vi "Intake_Joint_Set.vi"() -> ()   [LabVIEW 2018]
uses:
  Intake_Joint_Control_Type.ctl
  <vilib>/Rock Robotics/WPI/DriverStation/WPI_DriverStationRobotMode2.ctl
  Intake_Joint_Enum_States.ctl
  Global_Variables/Intake_Joint_Globals.vi
  Global_Variables/Robot_Global_Data.vi
  Global_Variables/Autonomous_Globals.vi
  Global_Variables/Intake_Disc_Globals.vi
panel:
  out "Cargo_Mode_for_Scoring":bool
  out "Cargo_Mode":bool
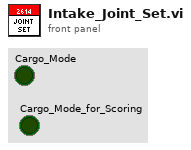
[diagram p1: front panel]
types:
  T1 = typedef "Intake_Joint_Control_Type.ctl" = enum16{"No_Op", "Manual_Joint_Up", "Manual_Joint_Down", "Manual_Position_Control", "Position_Control", "Position"}
  T2 = typedef "WPI_DriverStationRobotMode2.ctl" = enum16{"Autonomous Disabled", "Autonomous Enabled", "Teleop Disabled", "Teleop Enabled", "Disconnected", "Finish", "Test Disabled", "Test Enabled", "Emergency Stopped"}
  T3 = typedef "Intake_Joint_Enum_States.ctl" = enum16{"Current_Position", "High_Rocket_Hatch_Panel_Floor", "High_Rocket_Hatch_Panel", "Mid_Rocket_Hatch_Panel_Floor", "Mid_Rocket_Hatch_Panel", "Low_Rocket_Hatch_Panel", "Cargo_Ship_Hatch_Panel", "Loading_Station_Hatch_Panel", "Ground_Pickup_Hatch_Panel", "High_Rocket_Cargo", "Mid_Rocket_Cargo", "Low_Rocket_Cargo", "Cargo_Ship_Cargo", "Loading_Station_Cargo", "Ground_Pickup_Cargo", "Depot_Pickup_Cargo", "Stow_Cargo", "Get_Hatch"}
  T4 = typedef "Intake_Joint_Notifier.ctl" = cluster{"Intake_Joint_Control_Type":T1, "Manual_Joint_Up":bool, "Manual_Joint_Down":bool, "Low_Rocket":bool, "Mid_Rocket":bool, "High_Rocket":bool, "Cargo_Ship":bool, "Hatch_Floor":bool, "Cargo_Floor":bool, "HP_Hatch":bool, "HP_Cargo":bool, "Depot_Cargo":bool, "Stow":bool, "Intake_Mode":bool, "Set Position":T3, "Parameter_One":dbl, "Parameter_Two":dbl, "Parameter_Three":dbl, "Step":i32, "Joint_Notifier":refnum<notifier>}
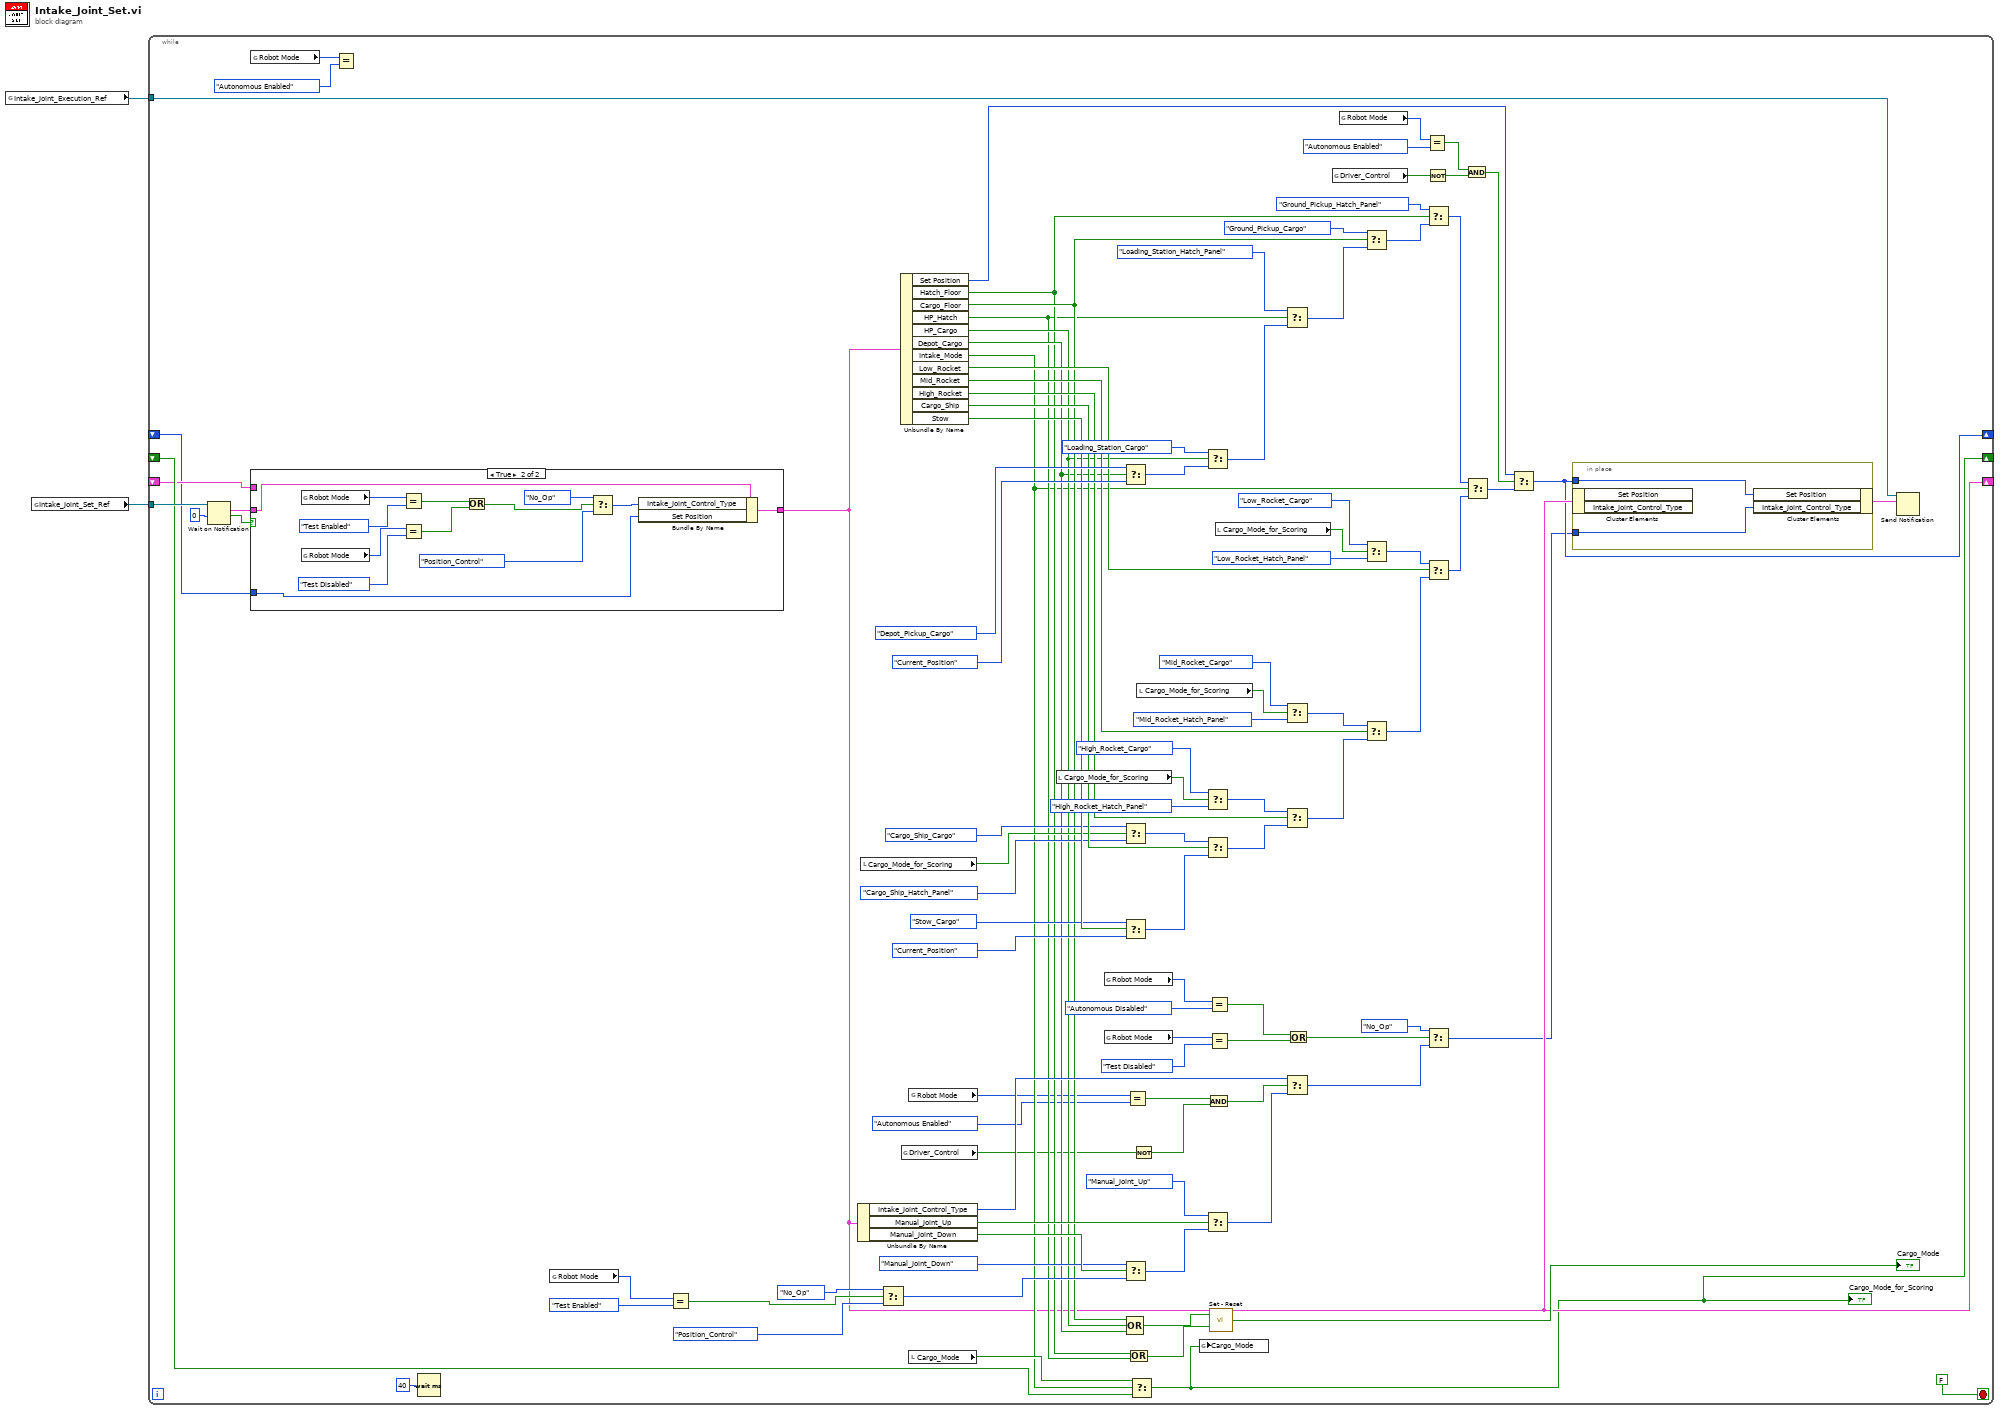
[diagram p0: block diagram]
diagram:
  n1 = global read "Intake_Joint_Globals.vi" "Intake_Joint_Execution_Ref"() -> (w1:refnum<notifier>)
  n2 = global read "Intake_Joint_Globals.vi" "Intake_Joint_Set_Ref"() -> (w2:refnum<notifier>)
  n3 = while {
    tunnel: w2 -> [w102]
    tunnel: w1 -> [w101]
    shift-right: [w23] -> _
    shift-left: _ -> [w36]
    shift-right: [w28] -> _
    shift-left: _ -> [w27]
    shift-right: [w25] -> _
    shift-left: _ -> [w24]
    stop <- FALSE stop-if-true
    n4 = Wait on Notification(notifier=w102, timeout in ms (-1)=0) -> (notification=w29:T4, timed out?=w26:bool)  [unwired: 2 in, 2 out]
    n5 = case shown="True" w26 {
      tunnel: w29 -> [w105 w117]
      tunnel: [w105 w118] -> w28
      tunnel: w27 -> [_ _]
      tunnel: w24 -> [_ w116]
      frame False {
      }
      frame True {
        n6 = global read "Robot_Global_Data.vi" "Robot Mode"() -> (w113:T2)
        n7 = global read "Robot_Global_Data.vi" "Robot Mode"() -> (w108:T2)
        n8 = Equal?(x=w113, y=WPI_DriverStationRobotMode2."Test Enabled") -> (x = y?=w110:bool)
        n9 = Equal?(x=w108, y=WPI_DriverStationRobotMode2."Test Disabled") -> (x = y?=w107:bool)
        n10 = Or(x=w110, y=w107) -> (x .or. y?=w106:bool)
        n11 = Select(t=Intake_Joint_Control_Type."No_Op", s=w106, f=Intake_Joint_Control_Type."Position_Control" ("Intake_Joint_Control_Type")) -> (s? t:f=w115:T1)
        n12 = Bundle By Name(cluster=w117, "Intake_Joint_Control_Type"=w115, "Set Position"=w116) -> (w118:T4)
      }
    }
    n13 = global read "Robot_Global_Data.vi" "Robot Mode"() -> (w100:T2)
    n14 = Equal?(x=w100, y=WPI_DriverStationRobotMode2."Autonomous Enabled") -> ()  [unwired: 1 out]
    n15 = Wait (ms)(milliseconds to wait=u32 40) -> ()  [unwired: 1 out]
    n16 = global read "Robot_Global_Data.vi" "Robot Mode"() -> (w89:T2)
    n17 = Equal?(x=w89, y=WPI_DriverStationRobotMode2."Test Enabled") -> (x = y?=w87:bool)
    n18 = Unbundle By Name(w28) -> ("Intake_Joint_Control_Type"=w98:T1, "Manual_Joint_Up"=w94:bool, "Manual_Joint_Down"=w93:bool)
    n19 = local read "Cargo_Mode_for_Scoring"() -> (w55:bool)
    n20 = Select(t=Intake_Joint_Control_Type."No_Op", s=w87, f=Intake_Joint_Control_Type."Position_Control" ("t")) -> (s? t:f=w88:T1)
    n21 = Unbundle By Name(w28) -> ("Set Position"=w31:T3, "Hatch_Floor"=w40:bool, "Cargo_Floor"=w45:bool, "HP_Hatch"=w39:bool, "HP_Cargo"=w44:bool, "Depot_Cargo"=w43:bool, "Intake_Mode"=w35:bool, "Low_Rocket"=w67:bool, "Mid_Rocket"=w66:bool, "High_Rocket"=w65:bool, "Cargo_Ship"=w64:bool, "Stow"=w63:bool)
    n22 = global read "Autonomous_Globals.vi" "Driver_Control"() -> (w17:bool)
    n23 = global read "Robot_Global_Data.vi" "Robot Mode"() -> (w15:T2)
    n24 = local read "Cargo_Mode"() -> (w42:bool)
    n25 = local read "Cargo_Mode_for_Scoring"() -> (w51:bool)
    n26 = global read "Robot_Global_Data.vi" "Robot Mode"() -> (w10:T2)
    n27 = global read "Robot_Global_Data.vi" "Robot Mode"() -> (w6:T2)
    n28 = Select(t=Intake_Joint_Enum_States."Depot_Pickup_Cargo", s=w43, f=Intake_Joint_Enum_States."Current_Position" ("Set Position")) -> (s? t:f=w80:T3)
    n29 = Select(t=Intake_Joint_Enum_States."Cargo_Ship_Cargo" ("Set Position"), s=w55, f=Intake_Joint_Enum_States."Cargo_Ship_Hatch_Panel") -> (s? t:f=w48:T3)
    n30 = Select(t=Intake_Joint_Enum_States."Stow_Cargo", s=w63, f=Intake_Joint_Enum_States."Current_Position" ("Set Position")) -> (s? t:f=w73:T3)
    n31 = Select(t=Intake_Joint_Control_Type."Manual_Joint_Down", s=w93, f=w88) -> (s? t:f=w96:T1)
    n32 = Equal?(x=w15, y=WPI_DriverStationRobotMode2."Autonomous Enabled") -> (x = y?=w18:bool)
    n33 = Compound Arithmetic op=OR(w45, w44, w43) -> (w46:bool)
    n34 = Compound Arithmetic op=OR(w40, w39) -> (w47:bool)
    n35 = Select(t=w42, s=w35, f=w36) -> (s? t:f=w23:bool)
    "Cargo_Mode_for_Scoring" <- w23
    n36 = Not(x=w17) -> (.not. x?=w16:bool)
    n37 = local read "Cargo_Mode_for_Scoring"() -> (w54:bool)
    n38 = global write "Intake_Disc_Globals.vi" "Cargo_Mode"(w23) -> ()
    n39 = Select(t=Intake_Joint_Enum_States."Loading_Station_Cargo", s=w44, f=w80) -> (s? t:f=w79:T3)
    n40 = Select(t=Intake_Joint_Enum_States."High_Rocket_Cargo" ("Set Position"), s=w51, f=Intake_Joint_Enum_States."High_Rocket_Hatch_Panel") -> (s? t:f=w49:T3)
    n41 = Select(t=w48, s=w64, f=w73) -> (s? t:f=w72:T3)
    n42 = Select(t=Intake_Joint_Control_Type."Manual_Joint_Up", s=w94, f=w96) -> (s? t:f=w95:T1)
    n43 = Equal?(x=w10, y=WPI_DriverStationRobotMode2."Autonomous Disabled") -> (x = y?=w9:bool)
    n44 = Equal?(x=w6, y=WPI_DriverStationRobotMode2."Test Disabled") -> (x = y?=w5:bool)
    n45 = And(x=w18, y=w16) -> (x .and. y?=w13:bool)
    n46 = call "Set - Reset.vi"("Reset"=w47, "Set"=w46) -> ("Output"=→"Cargo_Mode":bool)
    n47 = local read "Cargo_Mode_for_Scoring"() -> (w61:bool)
    n48 = Select(t=Intake_Joint_Enum_States."Loading_Station_Hatch_Panel", s=w39, f=w79) -> (s? t:f=w82:T3)
    n49 = Select(t=Intake_Joint_Enum_States."Mid_Rocket_Cargo" ("Set Position"), s=w54, f=Intake_Joint_Enum_States."Mid_Rocket_Hatch_Panel") -> (s? t:f=w52:T3)
    n50 = Select(t=w49, s=w65, f=w72) -> (s? t:f=w71:T3)
    n51 = Select(t=w98, s=w13, f=w95) -> (s? t:f=w12:T1)
    n52 = Or(x=w9, y=w5) -> (x .or. y?=w4:bool)
    n53 = global read "Autonomous_Globals.vi" "Driver_Control"() -> (w21:bool)
    n54 = global read "Robot_Global_Data.vi" "Robot Mode"() -> (w33:T2)
    n55 = Select(t=Intake_Joint_Enum_States."Ground_Pickup_Cargo", s=w45, f=w82) -> (s? t:f=w83:T3)
    n56 = Select(t=Intake_Joint_Enum_States."Low_Rocket_Cargo" ("Set Position"), s=w61, f=Intake_Joint_Enum_States."Low_Rocket_Hatch_Panel") -> (s? t:f=w58:T3)
    n57 = Select(t=w52, s=w66, f=w71) -> (s? t:f=w70:T3)
    n58 = Equal?(x=w33, y=WPI_DriverStationRobotMode2."Autonomous Enabled") -> (x = y?=w20:bool)
    n59 = Not(x=w21) -> (.not. x?=w22:bool)
    n60 = Select(t=Intake_Joint_Enum_States."Ground_Pickup_Hatch_Panel" ("Set Position"), s=w40, f=w83) -> (s? t:f=w84:T3)
    n61 = Select(t=w58, s=w67, f=w70) -> (s? t:f=w69:T3)
    n62 = Select(t=Intake_Joint_Control_Type."No_Op", s=w4, f=w12) -> (s? t:f=w11:T1)
    n63 = And(x=w20, y=w22) -> (x .and. y?=w19:bool)
    n64 = Select(t=w84, s=w35, f=w69) -> (s? t:f=w32:T3)
    n65 = Select(t=w31, s=w19, f=w32) -> (s? t:f=w25:T3)
    n66 = in-place {
      in-place-border: w11 -> [w120]
      in-place-border: w25 -> [w119]
      n67 = in-place-cluster #1(w28) -> ()  [unwired: 2 out]
      n68 = in-place-cluster #1("Set Position"=w119, "Intake_Joint_Control_Type"=w120) -> (w97:T4)
    }
    n69 = Send Notification(notification=w97, notifier=w101) -> ()  [unwired: 1 in, 2 out]
  }
